vi "specu1a 1.0.0 Open Pipe.vi"(3 "error in (no error)":errorcluster, 5 "Device Handle":i32) -> (0 "error out":errorcluster, 1 "Pipe Handle":i32, 2 "Device Handle out":i32)   [LabVIEW 2019]
uses:
  specu1a.dll
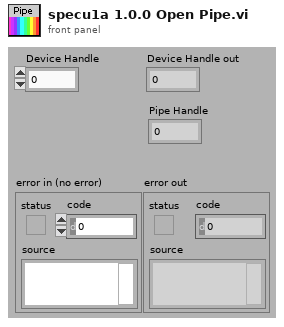
[diagram p1: front panel]
types:
  T1 = typedef "specu1a 1.0.0 Error codes.ctl" = enum16{"INVALID_HANDLE_VALUE", "USBDEV_SUCCESS", "USBDEV_INVALID_HANDLE", "USBDEV_UNSUCCESS", "USBDEV_INVALID_VALUE", "USBDEV_CHECK_NORMAL", "USBDEV_CHECK_INVALID", "USBDEV_CHECK_REMOVE", "USBDEV_CHECK_OTHER", "USBDEV_RESET_ERROR", "USBDEV_BULKSIZE_ERROR", "USBDEV_BULK_READ_ERROR", "USBDEV_BULK_NOT_UPDATED", "USBDEV_TIME_OVER_ERROR", "USBDEV_TIME_UNDER_ERROR", "USBDEV_TIME_SET_ERROR", "USBDEV_SET_GAIN_ERROR", "USBDEV_GET_TEMP_ERROR", "USBDEV_SET_TRIGGER_ERROR", "USBDEV_RW_EEP_ADDR_ERROR", "USBDEV_RW_EEP_SIZE_ERROR", "USBDEV_RW_EEP_OVER_ERROR", "USBDEV_RW_EEP_ERROR", "UNITID_PRODUCTID_CONFLICT", "UNKNOWN_ERROR"}
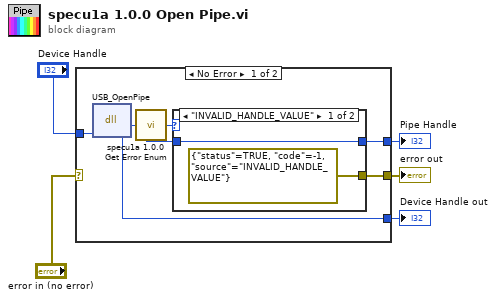
[diagram p0: block diagram]
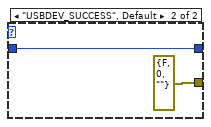
[diagram p2: hidden frame]
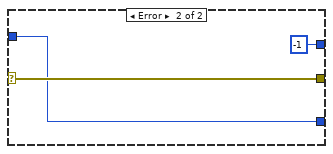
[diagram p3: hidden frame]
diagram:
  n1 = case shown="No Error" "error in (no error)" {
    selector: "error in (no error)" -> [_ w18]
    tunnel: "Device Handle" -> [w11 w17]
    tunnel: [w8 -1] -> w4
    tunnel: [w7 w17] -> w3
    tunnel: [w6 w18] -> w1
    frame No Error {
      n2 = dll-call lib="C:/Users/martzlab/Desktop/SIO 179/Nitrate/64/EvaluationSoftware/minispec labview/Hamamatsu Spectrometer Dll/specu1a.dll" fn="USB_OpenPipe" label="1.0.0 Open Pipe"("Device Handle"=w11) -> (w9:i32, "Device Handle"=w7:i32)  [unwired: 3 in, 2 out]
      n3 = call "specu1a 1.0.0 Get Error Enum.vi"("Error Code in"=w9) -> ("Specu1a 1.0.0 Error code out"=w10:T1)  [unwired: 4 in]
      n4 = case shown="\"INVALID_HANDLE_VALUE\"" w10 {
        tunnel: [w12 w14] -> w8
        tunnel: [errorcluster {"status"=TRUE, "code"=-1, "source"="INVALID_HANDLE_VALUE"} ("error out") errorcluster {"status"=FALSE, "code"=0, "source"=""} ("error out")] -> w6
        tunnel: w9 -> [w12 w14]
        frame "INVALID_HANDLE_VALUE" {
        }
        frame "USBDEV_SUCCESS", Default {
        }
      }
    }
    frame Error {
    }
  }
  "Device Handle out" <- w3
  "Pipe Handle" <- w4
  "error out" <- w1
